vi "Read Interface Configs.vi"(8 "error in (no error)":errorcluster, 10 "Device Ref in":T1 format="%.0x", 11 "Refnum in":T2) -> (0 "error out":errorcluster, 2 "Item Ref out":T1 format="%.0x", 3 "Refnum out":T2)   [LabVIEW 2021, in "Modbus Master System Explorer.lvlib"]
uses:
  Modbus Master System Explorer.lvlib
  <vilib>/NI VeriStand/Custom Device API/Custom Device Item Ref.ctl
  <vilib>/Utility/config.llb/Config Data RefNum.ctl
  Shared/Controls/Interface Type.ctl
  Shared/Constants.vi
  <vilib>/Utility/config.llb/Read Key (U32).vi
  <vilib>/NI VeriStand/Custom Device API/Set Item Property (U16).vi
  <vilib>/Utility/config.llb/Read Key (String).vi
  <vilib>/Utility/config.llb/Read Key (I32).vi
  <vilib>/Utility/config.llb/NI_LVConfig.lvlib
  <vilib>/NI VeriStand/Custom Device API/Custom Device API.lvlib
  Shared/Modbus Master Shared.lvlib
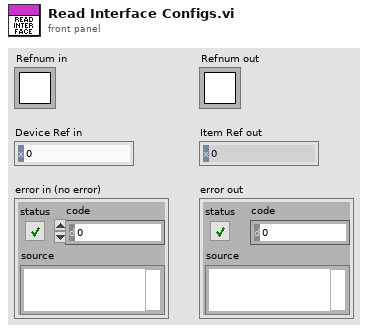
[diagram p1: front panel]
types:
  T1 = typedef "Custom Device API.lvlib/Custom Device Item Ref.ctl" = u64
  T2 = typedef "NI_LVConfig.lvlib/Config Data RefNum.ctl" = refnum<k1>
  T3 = typedef "Modbus Master Shared.lvlib/Interface Type.ctl" = enum16{"TCP Master", "Serial Master", "TCP Slave", "Serial Slave"}
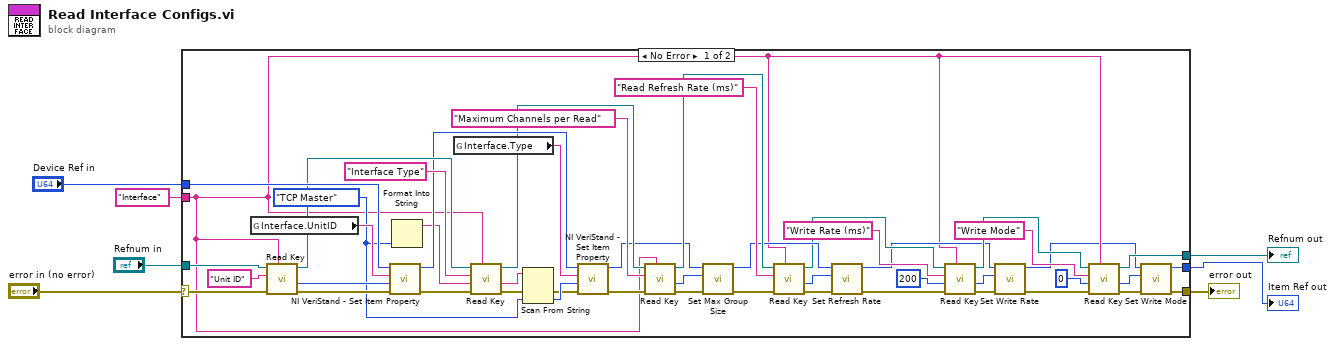
[diagram p0: block diagram]
diagram:
  n1 = case shown="No Error" "error in (no error)" {
    selector: "error in (no error)" -> [w53 w57]
    tunnel: "Device Ref in" -> [w55 w56]
    tunnel: "Refnum in" -> [w54 w58]
    tunnel: "Interface" ("section") -> [w16 _]
    tunnel: [w21 w58] -> w3
    tunnel: [w8 w57] -> w2
    tunnel: [w12 w56] -> w1
    frame No Error {
      w41 = Interface_Type."TCP Master" ("Interface Type")
      n2 = global read "Constants.vi" "Interface.UnitID"() -> (w46:string)
      n3 = call-poly <vilib>:"Read Key.vi"("section"=w16, "error in (no error)"=w53, "key"="Unit ID", "refnum"=w54) -> ("error out"=w51:errorcluster, "value"=w50:u32, "refnum out"=w48:T2)  [unwired: 4 in, 1 out]
      n4 = call-poly <vilib>:"NI VeriStand - Set Item Property.vi"("error in (no error)"=w51, "Value"=w50, "Property Name"=w46, "Item Ref in"=w55) -> ("error out"=w47:errorcluster, "Item Ref out"=w45:T1)  [unwired: 5 in, 1 out]
      n5 = Format Into String(w41) -> (resulting string=w40:string)  [unwired: 3 in, 1 out]
      n6 = global read "Constants.vi" "Interface.Type"() -> (w44:string)
      n7 = call-poly <vilib>:"Read Key.vi"("section"=w16, "error in (no error)"=w47, "default value"=w40, "key"="Interface Type", "refnum"=w48) -> ("error out"=w31:errorcluster, "value"=w43:string, "refnum out"=w39:T2)  [unwired: 3 in, 1 out]
      n8 = Scan From String(input string=w43, error in=w31, default 1=w41) -> (error out=w30:errorcluster, output 1=w42:T3)  [unwired: 2 in, 2 out]
      n9 = call-poly <vilib>:"NI VeriStand - Set Item Property.vi"("error in (no error)"=w30, "Value"=w42, "Property Name"=w44, "Item Ref in"=w45) -> ("error out"=w29:errorcluster, "Item Ref out"=w33:T1)  [unwired: 5 in, 1 out]
      n10 = call-poly <vilib>:"Read Key.vi"("section"=w16, "error in (no error)"=w29, "key"="Maximum Channels per Read", "refnum"=w39) -> ("error out"=w28:errorcluster, "value"=w37:i32, "refnum out"=w36:T2)  [unwired: 4 in, 1 out]
      n11 = call "Set Max Group Size.vi"("error in (no error)"=w28, "Value"=w37, "Item Ref in"=w33) -> ("error out"=w27:errorcluster, "Item Ref out"=w32:T1)  [unwired: 7 in]
      n12 = call-poly <vilib>:"Read Key.vi"("section"=w16, "error in (no error)"=w27, "key"="Read Refresh Rate (ms)", "refnum"=w36) -> ("error out"=w26:errorcluster, "value"=w34:i32, "refnum out"=w23:T2)  [unwired: 4 in, 1 out]
      n13 = call "Set Refresh Rate.vi"("error in (no error)"=w26, "Value"=w34, "Item Ref in"=w32) -> ("error out"=w17:errorcluster, "Item Ref out"=w19:T1)  [unwired: 7 in]
      n14 = call-poly <vilib>:"Read Key.vi"("section"=w16, "error in (no error)"=w17, "default value"=200, "key"="Write Rate (ms)", "refnum"=w23) -> ("error out"=w18:errorcluster, "value"=w15:i32, "refnum out"=w22:T2)  [unwired: 3 in, 1 out]
      n15 = call "Set Write Rate.vi"("error in (no error)"=w18, "Value"=w15, "Item Ref in"=w19) -> ("error out"=w11:errorcluster, "Item Ref out"=w13:T1)  [unwired: 7 in]
      n16 = call-poly <vilib>:"Read Key.vi"("section"=w16, "error in (no error)"=w11, "default value"=0, "key"="Write Mode", "refnum"=w22) -> ("error out"=w9:errorcluster, "value"=w14:u32, "refnum out"=w21:T2)  [unwired: 3 in, 1 out]
      n17 = call "Set Write Mode.vi"("error in (no error)"=w9, "Write Mode"=w14, "Item Ref in"=w13) -> ("error out"=w8:errorcluster, "Item Ref out"=w12:T1)  [unwired: 7 in]
    }
    frame Error {
    }
  }
  "Refnum out" <- w3
  "error out" <- w2
  "Item Ref out" <- w1
